vi "InitGPX.vi"(8 "error in (no error)":errorcluster) -> (0 "error out":errorcluster)   [LabVIEW 2015, in "ESLSCDLL.lvlib"]
uses:
  ESLSCDLL.lvlib
  Globals.vi
  ESLSCDLL.dll
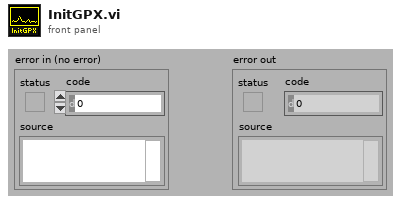
[diagram p1: front panel]
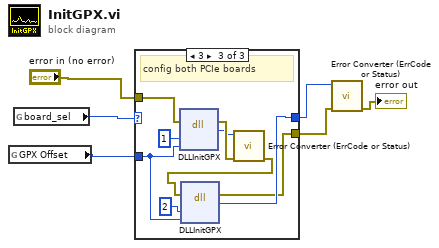
[diagram p0: block diagram]
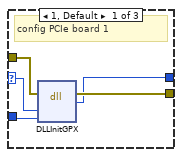
[diagram p2: hidden frame]
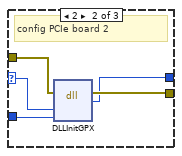
[diagram p3: hidden frame]
diagram:
  n1 = global read "Globals.vi" "GPX Offset"() -> (w1:u32)
  n2 = global read "Globals.vi" "board_sel"() -> (w2:u32)
  n3 = case shown="3" w2 {
    selector: w2 -> [w11 w16 _]
    tunnel: w1 -> [w10 w15 w25]
    tunnel: "error in (no error)" -> [w9 w14 w22]
    tunnel: [w8 w13 w17] -> w4
    tunnel: [w7 w12 w18] -> w3
    frame 1, Default {
      # "config PCIe board 1"
      n4 = dll-call lib="C:/Users/flori/Nextcloud/Dokumente/Stresing/Windows/lv64/board.vis/ESLSCDLL.dll" fn="DLLInitGPX" ("lwlscdll.dll:DLLWriteLongS0")(error in=w9, "drv"=w11, "delay"=w10) -> (error out=w8:errorcluster, "es_status_codes"=w7:i32)  [unwired: 4 in, 1 out]
    }
    frame 2 {
      # "config PCIe board 2"
      n5 = dll-call lib="C:/Users/flori/Nextcloud/Dokumente/Stresing/Windows/lv64/board.vis/ESLSCDLL.dll" fn="DLLInitGPX" ("lwlscdll.dll:DLLWriteLongS0")(error in=w14, "drv"=w16, "delay"=w15) -> (error out=w13:errorcluster, "es_status_codes"=w12:i32)  [unwired: 4 in, 1 out]
    }
    frame 3 {
      # "config both PCIe boards"
      n6 = dll-call lib="C:/Users/flori/Nextcloud/Dokumente/Stresing/Windows/lv64/board.vis/ESLSCDLL.dll" fn="DLLInitGPX" ("lwlscdll.dll:DLLWriteLongS0")(error in=w22, "drv"=u32 1, "delay"=w25) -> (error out=w21:errorcluster, "es_status_codes"=w20:i32)  [unwired: 4 in, 1 out]
      n7 = call "Error Converter (ErrCode or Status).vi"("error in (no error)"=w21, "error code"=w20) -> ("error out"=w19:errorcluster)  [unwired: 9 in]
      n8 = dll-call lib="C:/Users/flori/Nextcloud/Dokumente/Stresing/Windows/lv64/board.vis/ESLSCDLL.dll" fn="DLLInitGPX" ("lwlscdll.dll:DLLWriteLongS0")(error in=w19, "drv"=u32 2, "delay"=w25) -> (error out=w17:errorcluster, "es_status_codes"=w18:i32)  [unwired: 4 in, 1 out]
    }
  }
  n9 = call "Error Converter (ErrCode or Status).vi"("error in (no error)"=w4, "error code"=w3) -> ("error out"=→"error out":errorcluster)  [unwired: 9 in]
